vi "Data Global.vi"(7 "Operate":T2=enum."Read", 8 "error in (no error)":errorcluster caption="Error In", 9 "Data In":map{string, T1}(c390), 10 "Data":map{string, string}(c390), 11 "Name":string) -> (0 "error out":errorcluster caption="Error Out", 1 "x-y":u32, 2 "Project":string, 3 "Data Out":map{string, T1}(c390))   [LabVIEW 2020]
uses:
  Data Global Mode.ctl
  SDQ Data Type.ctl
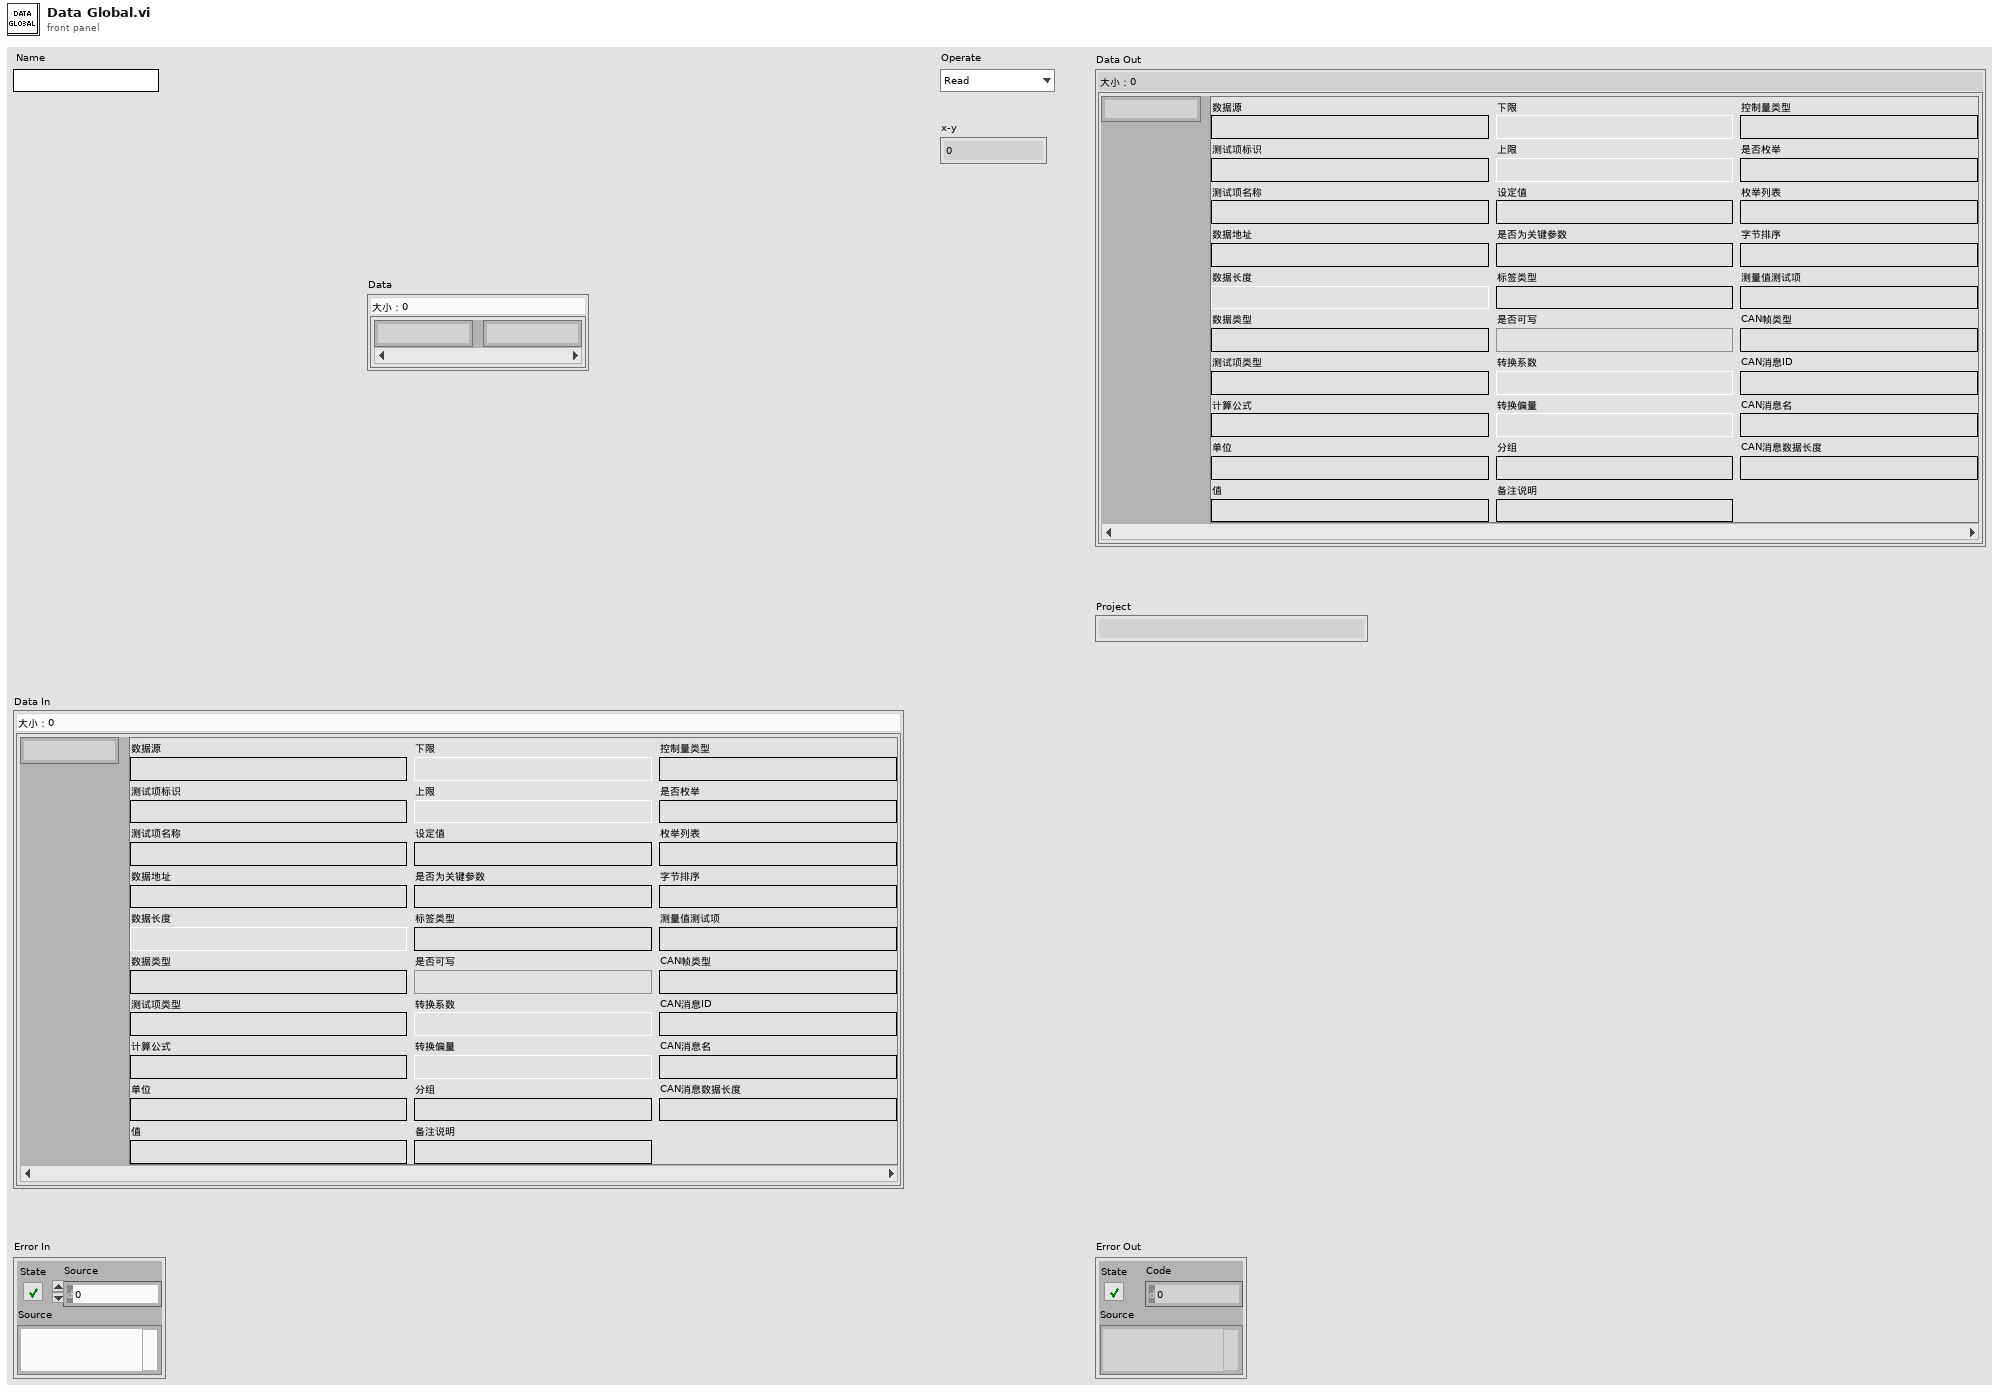
[diagram p1: front panel]
types:
  T1 = typedef "SDQ Data Type.ctl" = cluster{"CAN Length":string, "CAN Name":string, "CAN ID":string, "CAN Type":string, "Test Item":string, "Byte Order":string, "Instruction":string, "Control Type":string, "Group":string, "Offset":dbl, "Coefficient":dbl, "Write Enable":bool, "Lable Type":string, "Key?":string, "Set Value":string, "Upper":dbl, "Lower":dbl, "Unit":string, "Formula":string, "Test Item Type":string, "Length":i32, "Address":string, "Name":string, "Identifier":string, "Data Type":string, "Enumerate?":string, "Enumerate List":string, "Data":string, "Source":string}
  T2 = typedef "Data Global Mode.ctl" = enum16{"Init", "Read", "Write", "Write Data", "Load"}
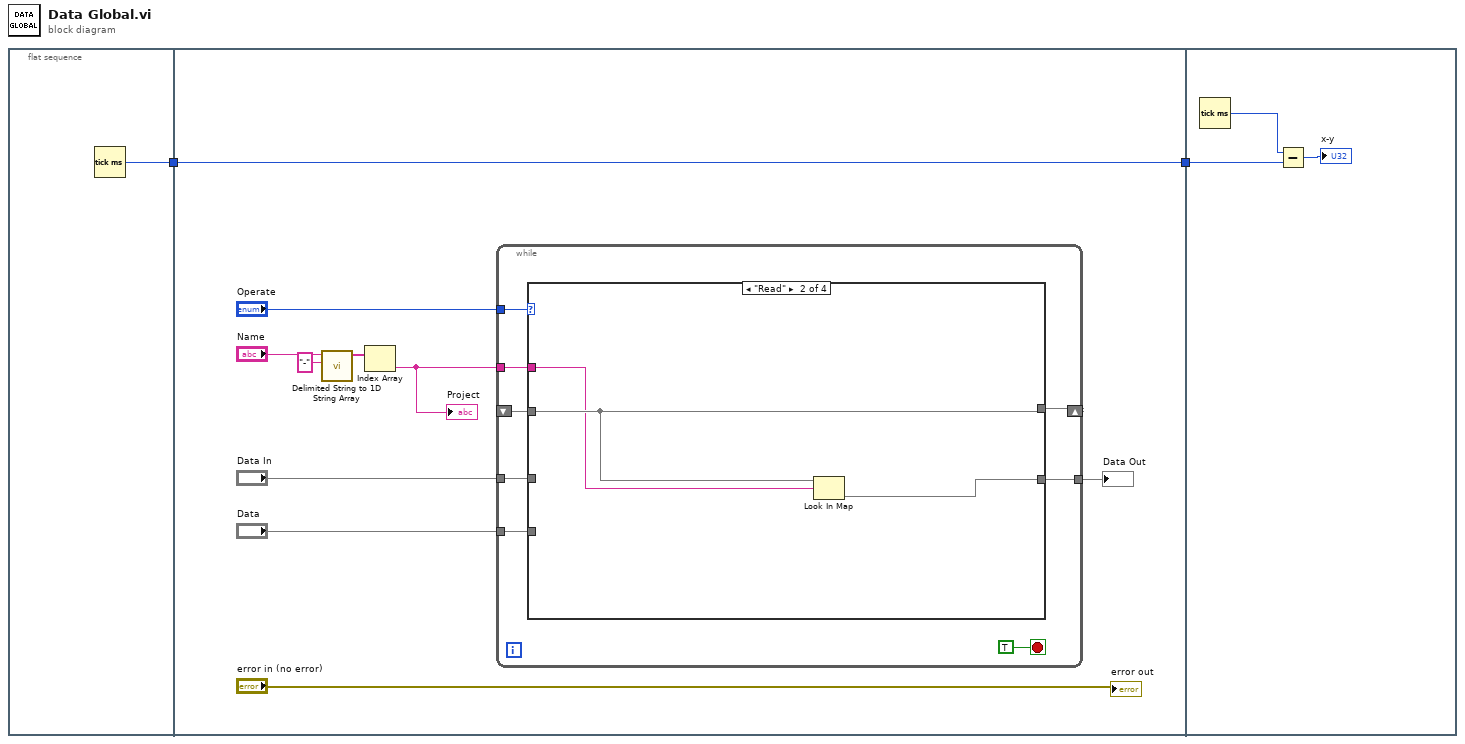
[diagram p0: block diagram]
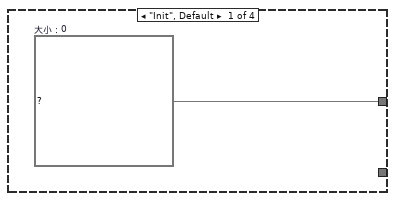
[diagram p2: hidden frame]
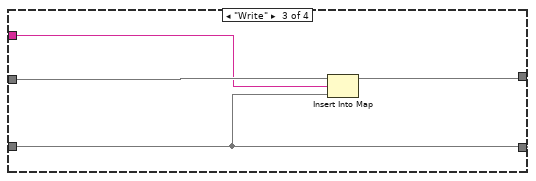
[diagram p3: hidden frame]
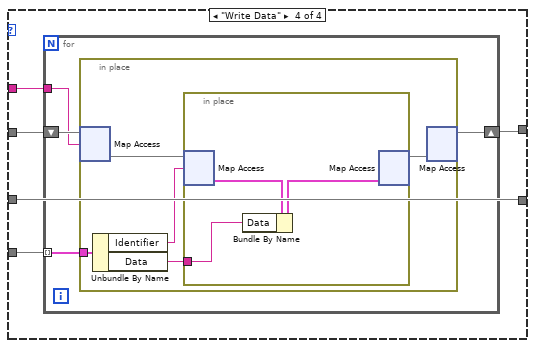
[diagram p4: hidden frame]
diagram:
  n1 = flat-sequence {
    tunnel: [w3] -> w1
    tunnel: [w5] -> w2
    tunnel: w1 -> [w5]
    tunnel: w2 -> [w48]
    frame #0 {
      n2 = Tick Count (ms)() -> (millisecond timer value=w3:u32)
    }
    frame #1 {
      n3 = call <vilib>:"Delimited String to 1D String Array.vi"("delimiter"="-", "delimited string"="Name") -> ("string array"=w7:string[])  [unwired: 9 in]
      n4 = Index Array(array=w7) -> (element=w6:string)  [unwired: 1 in]
      "Project" <- w6
      n5 = while {
        tunnel: "Operate" -> [w21]
        tunnel: w6 -> [w19]
        shift-right: [w18] -> _
        shift-left: _ -> [w17]
        tunnel: "Data In" -> [w16]
        tunnel: [w15] -> w11
        tunnel: "Data" -> [w14]
        stop <- TRUE stop-if-true
        n6 = case shown="\"Read\"" w21 {
          tunnel: w19 -> [_ w24 w27 w33]
          tunnel: [w22 w25 w28 w34] -> w18
          tunnel: w17 -> [_ w25 w29 w31]
          tunnel: w16 -> [_ _ w26 w32]
          tunnel: [_ w23 w26 w32] -> w15
          tunnel: w14 -> [_ _ _ w30]
          frame "Init", Default {
            w22 = map{string, map{string, T1}} {}  # 大小：0
          }
          frame "Read" {
            n7 = Look In Map(map=w25, key=w24) -> (value=w23:map{string, T1})  [unwired: 1 in, 1 out]
          }
          frame "Write" {
            n8 = Insert Into Map(map in=w29, key=w27, value=w26) -> (map out=w28:map{string, map{string, T1}})  [unwired: 2 out]
          }
          frame "Write Data" {
            n9 = for {
              tunnel: w33 -> [w37]
              shift-right: [w35] -> w34
              shift-left: w31 -> [w38]
              tunnel: w30 -> [w36] mode=indexing
              n10 = in-place {
                in-place-border: w36 -> [w42]
                n11 = in-place-map #1(w38, w37) -> (w43:map{string, T1})  [unwired: 1 in, 1 out]
                n12 = Unbundle By Name(w42) -> ("Identifier"=w41:string, "Data"=w40:string)
                n13 = in-place {
                  in-place-border: w40 -> [w44]
                  n14 = in-place-map #2(w43, w41) -> (w46:T1)  [unwired: 1 in, 1 out]
                  n15 = Bundle By Name(cluster=w46, "Data"=w44) -> (w45:T1)
                  n16 = in-place-map #2(w45) -> (w39:map{string, T1})  [unwired: 1 in, 2 out]
                }
                n17 = in-place-map #1(w39) -> (w35:map{string, map{string, T1}})  [unwired: 1 in, 2 out]
              }
            }
          }
        }
      }
      "Data Out" <- w11
      "error out" <- "error in (no error)"
    }
    frame #2 {
      n18 = Tick Count (ms)() -> (millisecond timer value=w49:u32)
      n19 = Subtract(x=w49, y=w48) -> (x-y=→"x-y":u32)
    }
  }
